vi "paths.vi"() -> (0 "Journal Folder":path, 1 "Controlsettings2":path, 2 "Journal Templates":path, 3 "PubAppData":path)   [LabVIEW 2013, in "main.lvlib"]
uses:
  main.lvlib
  <vilib>/Utility/sysdir.llb/System Directory Type.ctl
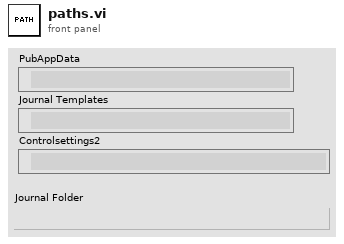
[diagram p1: front panel]
types:
  T1 = typedef "System Directory Type.ctl" = i32
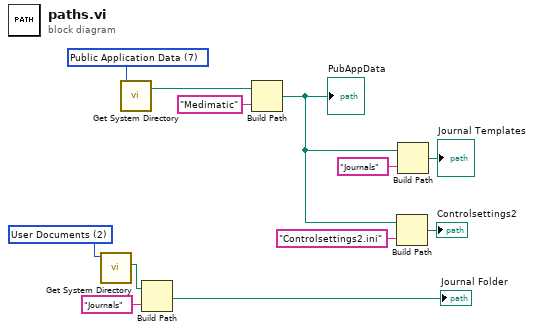
[diagram p0: block diagram]
diagram:
  w3 = T1 2 items=["User Home"=0, "User Desktop"=1, "User Documents"=2, "User Application Data"=3, "User Preferences"=4, "User Temporary"=5, "Public Documents"=6, "Public Application Data"=7, "Public Preferences"=8, "Public Cache"=13, "System Core Libraries"=9, "System Installed Libraries"=10, "Application Files"=11, "Boot Volume Root"=12] ("system directory type")
  w12 = T1 7 items=["User Home"=0, "User Desktop"=1, "User Documents"=2, "User Application Data"=3, "User Preferences"=4, "User Temporary"=5, "Public Documents"=6, "Public Application Data"=7, "Public Preferences"=8, "Public Cache"=13, "System Core Libraries"=9, "System Installed Libraries"=10, "Application Files"=11, "Boot Volume Root"=12] ("system directory type")
  n1 = call <vilib>:"Get System Directory.vi"("system directory type"=w3) -> ("system directory"=w2:path)  [unwired: 10 in]
  n2 = call <vilib>:"Get System Directory.vi"("system directory type"=w12) -> ("system directory"=w11:path)  [unwired: 10 in]
  n3 = Build Path(base path=w2, name or relative path="Journals") -> (appended path=→"Journal Folder":path)
  n4 = Build Path(base path=w11, name or relative path="Medimatic") -> (appended path=w7:path)
  "PubAppData" <- w7
  n5 = Build Path(base path=w7, name or relative path="Controlsettings2.ini") -> (appended path=→"Controlsettings2":path)
  n6 = Build Path(base path=w7, name or relative path="Journals") -> (appended path=→"Journal Templates":path)
